vi "Computer name.vi"(6 "cmd":enum16{"Load Name", "Read Name"}(ring), 8 "error in (no error)":errorcluster) -> (0 "error out":errorcluster, 3 "Computer name":string)   [LabVIEW 2015]
panel:
  in  "command line":string="netstat"
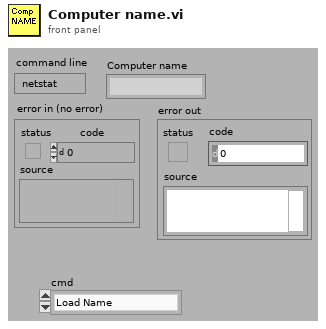
[diagram p1: front panel]
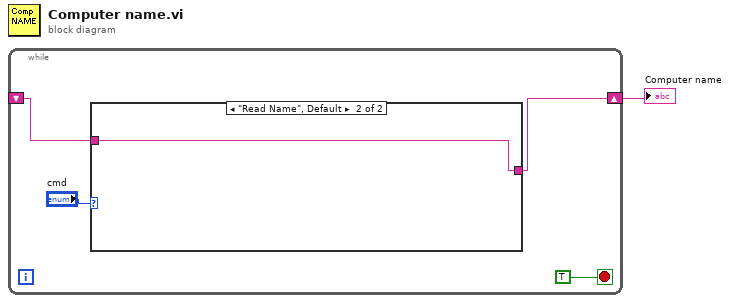
[diagram p0: block diagram]
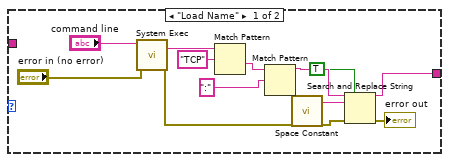
[diagram p2: hidden frame]
diagram:
  n1 = while {
    shift-right: [w3] -> w1
    shift-left: _ -> [w2]
    stop <- TRUE stop-if-true
    n2 = case shown="\"Read Name\", Default" "cmd" {
      tunnel: [w6 w18] -> w3
      tunnel: w2 -> [_ w18]
      frame "Load Name" {
        n3 = call <vilib>:"System Exec.vi"("error in (no error)"="error in (no error)", "command line"="command line") -> ("error out"=w7:errorcluster, "standard output"=w16:string)  [unwired: 6 in, 2 out]
        n4 = Match Pattern(string=w16, regular expression="TCP") -> (after substring=w14:string)  [unwired: 1 in, 3 out]
        n5 = Match Pattern(string=w14, regular expression=":") -> (before substring=w11:string)  [unwired: 1 in, 3 out]
        n6 = call <vilib>:"Space Constant.vi"() -> ("String"=w12:string)
        n7 = Search and Replace String(replace all?=TRUE ("replace all? (F)"), input string=w11, search string=w12, error in=w7) -> (result string=w6:string, error out=→"error out":errorcluster)  [unwired: 4 in, 2 out]
      }
      frame "Read Name", Default {
      }
    }
  }
  "Computer name" <- w1
